vi "借助分隔栏调整控件尺寸.vi"() -> ()   [LabVIEW 2010]
doc: "本VI是为《我和LabVIEW》一书编写的示例。\n关于本书的介绍请参考网页：\nhttp://ruanqizhen.spaces.live.com/blog/cns!5852D4F797C53FB6!4310.entry"
panel:
  out "水箱":dbl(slide) scale=0.0..10.0
  out "油箱":dbl(slide) scale=0.0..10.0
  out "波形图":dbl[](graph)
  in  "信息":string
  in  "停止":bool
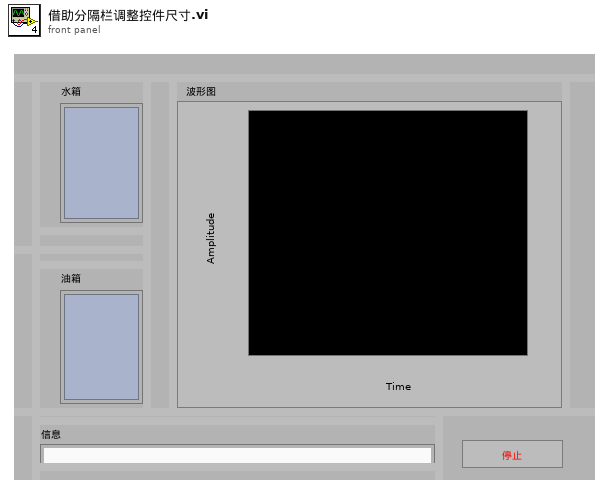
[diagram p1: front panel]
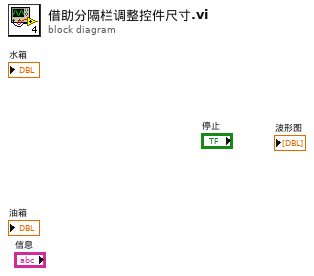
[diagram p0: block diagram]
diagram:
